vi "teleop aimer.vi"(10 "velocity":dbl, 11 "Distance":dbl) -> (0 "Aim Possible?":bool, 3 "Target Vert Angle":dbl)   [LabVIEW 2015]
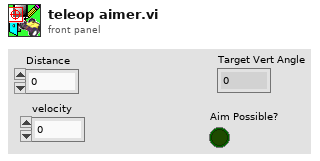
[diagram p1: front panel]
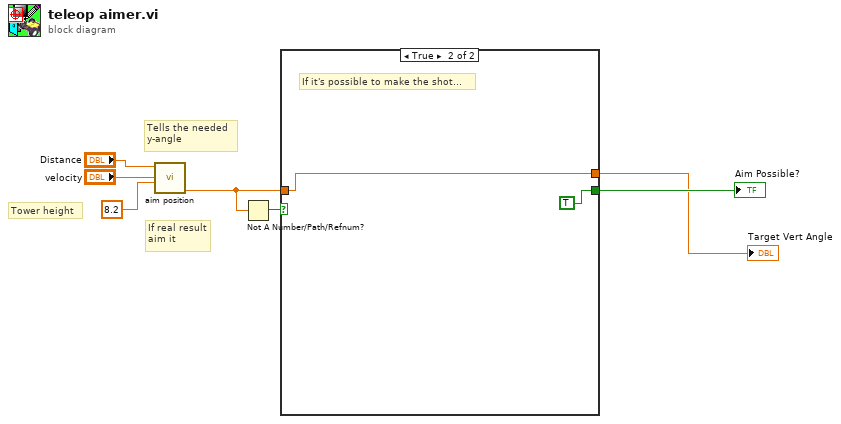
[diagram p0: block diagram]
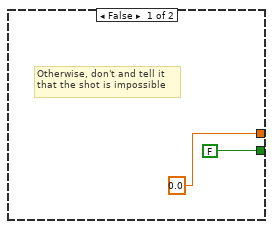
[diagram p2: hidden frame]
diagram:
  # "Tells the needed \ny-angle"
  # "If real result\naim it"
  # "Tower height"
  n1 = call "aim position.vi"("height"=8.2, "velocity"="velocity", "distance"="Distance") -> ("angle"=w3:dbl)  [unwired: 5 in, 1 out]
  n2 = Not A Number/Path/Refnum?(number/path/refnum=w3) -> (NaN/Path/Refnum?=w4:bool)
  n3 = case shown="True" w4 {
    tunnel: w3 -> [_ w10]
    tunnel: [FALSE TRUE] -> w2
    tunnel: [0.0 w10] -> w1
    frame False {
      # "Otherwise, don't and tell it \nthat the shot is impossible"
    }
    frame True {
      # "If it's possible to make the shot..."
    }
  }
  "Target Vert Angle" <- w1
  "Aim Possible?" <- w2
